vi "Sensor Module.vi"(8 "error in":errorcluster) -> (0 "error out":errorcluster)   [LabVIEW 2018, in "Sensor Interface.lvlib"]
doc: "This is the top level of the sensor module (a free running module of the Car WAsh simulator). \n\nIt is closed using a user event. It communicates with the other modules using a queue based API which has comms modules that can be swapped if required."
uses:
  Sensor Interface.lvlib
  Private Controls/Module Action.ctl
  Private Controls/Module Data Cluster.ctl
  Public Controls/Sensor Cluster.ctl
  Public Controls/Sensor Array.ctl
panel:
  in  "Settings":T1=[{"Variant"=variant(enum16{"Entry", "Station 1", "Station 2", "Station 3", "Exit", "Out of Position"} enum."Entry")}, {"Variant"=variant(enum16{"Entry", "Station 1", "Station 2", "Station 3", "Exit", "Out of Position"} enum."Station 1")}, {"Variant"=variant(enum16{"Entry", "Station 1", "Station 2", "Station 3", "Exit", "Out of Position"} enum."Station 1")}, {"Variant"=variant(enum16{"Entry", "Station 1", "Station 2", "Station 3", "Exit", "Out of Position"} enum."Station 2")}, {"Variant"=variant(enum16{"Entry", "Station 1", "Station 2", "Station 3", "Exit", "Out of Position"} enum."Station 2")}, {"Variant"=variant(enum16{"Entry", "Station 1", "Station 2", "Station 3", "Exit", "Out of Position"} enum."Station 2")}, {"Variant"=variant(enum16{"Entry", "Station 1", "Station 2", "Station 3", "Exit", "Out of Position"} enum."Station 2")}, {"Variant"=variant(enum16{"Entry", "Station 1", "Station 2", "Station 3", "Exit", "Out of Position"} enum."Station 3")}, {"Variant"=variant(enum16{"Entry", "Station 1", "Station 2", "Station 3", "Exit", "Out of Position"} enum."Station 3")}, {"Variant"=variant(enum16{"Entry", "Station 1", "Station 2", "Station 3", "Exit", "Out of Position"} enum."Exit")}]
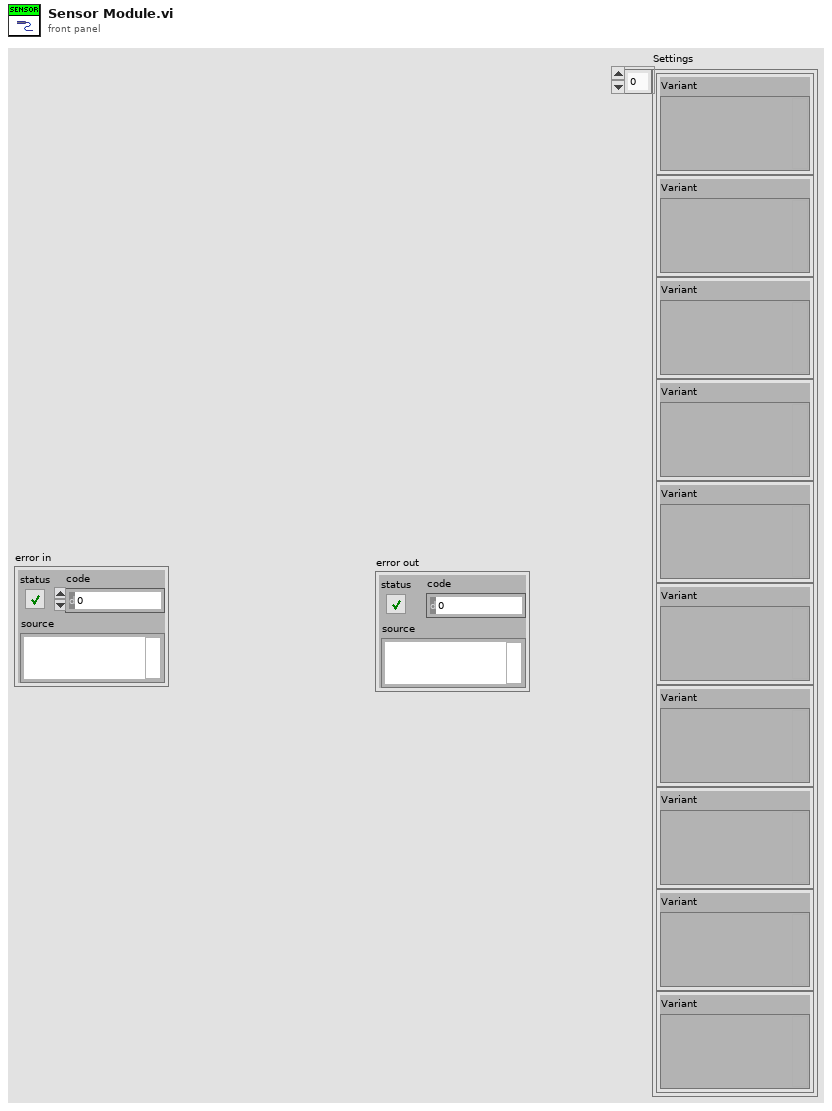
[diagram p1: front panel]
types:
  T1 = typedef "Sensor Interface.lvlib/Sensor Array.ctl" = T2[]
  T2 = typedef "Sensor Interface.lvlib/Sensor Cluster.ctl" = cluster{"Variant":variant}
  T3 = typedef "Sensor Interface.lvlib/Module Data Cluster.ctl" = cluster{"Variant":variant, "action":T4}
  T4 = typedef "Sensor Interface.lvlib/Module Action.ctl" = enum16{"error", "exit", "init", "Start Sim", "Update Position"}
  T5 = cluster{"Variant":variant, "action":enum16{"error", "exit", "init"}}
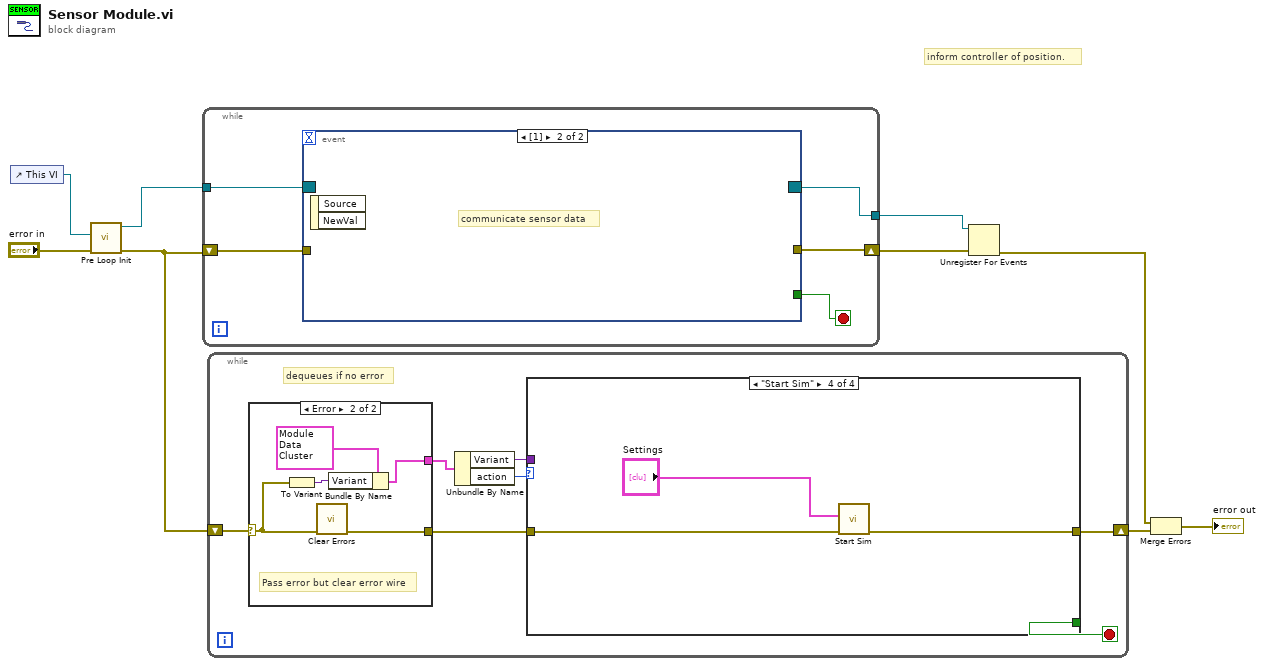
[diagram p0: block diagram]
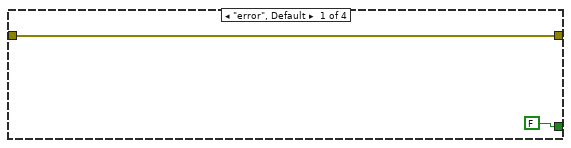
[diagram p2: hidden frame]
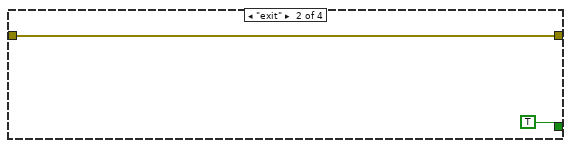
[diagram p3: hidden frame]
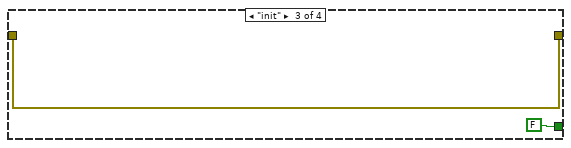
[diagram p4: hidden frame]
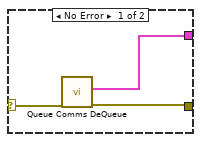
[diagram p5: hidden frame]
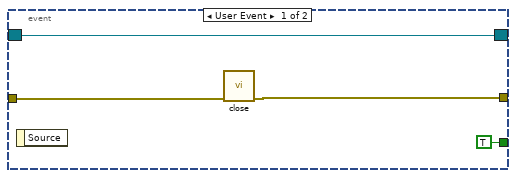
[diagram p6: hidden frame]
diagram:
  # "inform controller of position."
  n1 = control-ref of="This VI"() -> (w9:refnum<vi>)
  n2 = call "Pre Loop Init.vi"("error in"="error in", "Ref In"=w9) -> ("error out"=w6:errorcluster, "Event Registration Refnum"=w8:refnum<event-registration>)  [unwired: 8 in]
  n3 = while {
    shift-right: [w13] -> w5
    shift-left: w6 -> [w14]
    tunnel: w8 -> [w12]
    tunnel: [w10] -> w4
    stop <- w11 stop-if-true
    n4 = event shown="[1]" {
      selector: w12 -> [w15 _]
      dyn-events: [w15 _] -> w10
      timeout: _ -> [_ _]
      tunnel: w14 -> [w18 _]
      tunnel: [w17 _] -> w13
      tunnel: [TRUE _] -> w11
      event User Event {
        n5 = event-data() -> ()  [unwired: 1 in, 1 out]
        n6 = call "close.vi"("error in"=w18) -> ("error out"=w17:errorcluster)  [unwired: 10 in]
      }
      event #1 (no event record) {
        # "communicate sensor data"
        n7 = event-data() -> ()  [unwired: 1 in, 2 out]
      }
    }
  }
  n8 = while {
    shift-right: [w21] -> w3
    shift-left: w6 -> [w25]
    stop <- w19 stop-if-true
    # "dequeues if no error"
    n9 = case shown="Error" w25 {
      selector: w25 -> [w37 w42]
      tunnel: [w36 w38] -> w24
      tunnel: [w35 w41] -> w20
      frame No Error {
        n10 = call "Queue Comms DeQueue.vi"("error in"=w37) -> ("error out"=w35:errorcluster, "element"=w36:T5)  [unwired: 9 in]
      }
      frame Error {
        # "Pass error but clear error wire"
        n11 = To Variant(anything=w42) -> (Variant=w39:variant)
        n12 = call <vilib>:"Clear Errors.vi"("error in (no error)"=w42) -> ("error out"=w41:errorcluster)  [unwired: 5 in, 1 out]
        n13 = Bundle By Name(cluster=T3 {"Variant"=variant, "action"=enum."error"} ("element"), "Variant"=w39) -> (w38:T3)
      }
    }
    n14 = Unbundle By Name(w24) -> ("Variant"=w22:variant, "action"=w23:T4)
    n15 = case shown="\"Start Sim\"" w23 {
      tunnel: w22 -> [_ _ _ _]
      tunnel: [w27 w28 w31 w32] -> w21
      tunnel: w20 -> [w27 w28 w31 w33]
      tunnel: [FALSE TRUE FALSE _] -> w19
      frame "error", Default {
      }
      frame "exit" {
      }
      frame "init" {
      }
      frame "Start Sim" {
        n16 = call "Start Sim.vi"("error in"=w33, "data"="Settings") -> ("error out"=w32:errorcluster)  [unwired: 9 in]
      }
    }
  }
  n17 = Unregister For Events(event registration refnum=w4, error in=w5) -> (error out=w1:errorcluster)
  n18 = Merge Errors(w1, w3) -> (→"error out":errorcluster)
